vi "Parse Items To Analyze.vi"(8 "error in":errorcluster, 11 "ItemsToAnalyze Element":refnum<k20>) -> (0 "error out":errorcluster, 2 "Items To Analyze":cluster{"Item Path":path, "Removed?":bool}[](array[cluster]))   [LabVIEW 2020]
uses:
  <vilib>/xml/Close Reference(Node).vi
  <vilib>/xml/NI_XML.lvlib
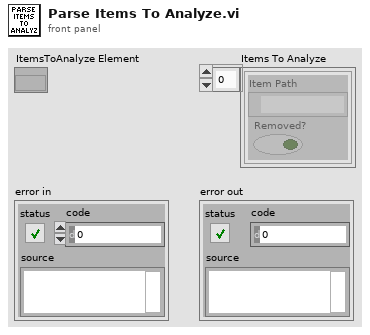
[diagram p1: front panel]
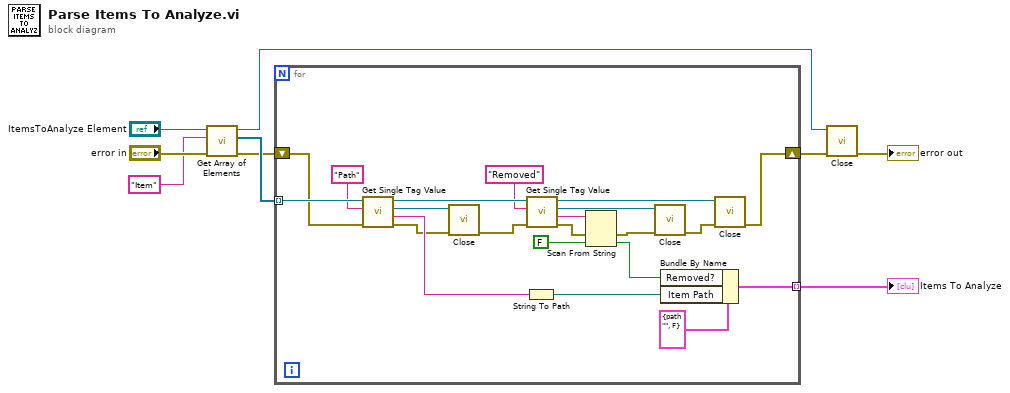
[diagram p0: block diagram]
diagram:
  n1 = call <vilib>:"Get Array of Elements.vi"("error in (no error)"="error in", "Tag Name"="Item", "Refnum in"="ItemsToAnalyze Element") -> ("error out"=w3:errorcluster, "Array Of Elements"=w4:refnum<k20>[], "Refnum out"=w5:refnum<k20>)  [unwired: 6 in]
  n2 = for {
    tunnel: w4 -> [w29] mode=indexing
    shift-right: [w21] -> w8
    shift-left: w3 -> [w28]
    tunnel: [w20] -> w9 mode=indexing
    n3 = call <vilib>:"Get Single Tag Value.vi"("Error In"=w28, "Tag Name"="Path", "Element In"=w29) -> ("Error Out"=w14:errorcluster, "Tag Value"=w16:string, "Tag Reference"=w15:refnum<k20>, "Element Out"=w27:refnum<k20>)  [unwired: 5 in]
    n4 = call-poly <vilib>:"Close.vi"("error in (no error)"=w14, "node"=w15) -> ("error out"=w10:errorcluster)  [unwired: 7 in]
    n5 = String To Path(string=w16) -> (path=w26:path)
    n6 = call <vilib>:"Get Single Tag Value.vi"("Error In"=w10, "Tag Name"="Removed", "Element In"=w27) -> ("Error Out"=w25:errorcluster, "Tag Value"=w17:string, "Tag Reference"=w13:refnum<k20>, "Element Out"=w22:refnum<k20>)  [unwired: 5 in]
    n7 = Scan From String(input string=w17, error in=w25, default 1=FALSE) -> (error out=w12:errorcluster, output 1=w23:bool)  [unwired: 2 in, 2 out]
    n8 = call-poly <vilib>:"Close.vi"("error in (no error)"=w12, "node"=w13) -> ("error out"=w11:errorcluster)  [unwired: 7 in]
    n9 = Bundle By Name(cluster=cluster{"Item Path":path, "Removed?":bool} {"Item Path"=path "", "Removed?"=FALSE} ("Cluster"), "Removed?"=w23, "Item Path"=w26) -> (w20:cluster{"Item Path":path, "Removed?":bool})
    n10 = call-poly <vilib>:"Close.vi"("error in (no error)"=w11, "node"=w22) -> ("error out"=w21:errorcluster)  [unwired: 7 in]
  }
  "Items To Analyze" <- w9
  n11 = call-poly <vilib>:"Close.vi"("error in (no error)"=w8, "node"=w5) -> ("error out"=→"error out":errorcluster)  [unwired: 7 in]
